vi "HAPS_PhaseGainSweep_Preamp.vi"() -> ()   [LabVIEW 2023, in "HAPS.lvlib"]
uses:
  HAPS.lvlib
  HAPS_SerialPort.ctl
  MCU_Function.ctl
  set_ele.ctl
  HAPS_MCU_ELE_Func.ctl
  R_S/R_S.lvlib
panel:
  out "dup path":path
  out "Phase_step":i32
  out "Gain_step":i32
  out "channel":i32
  out "chain_id":i32
  out "group":i32
  out "array_id":i32
  in  "Gain_Start_Step":i32=16
  in  "Phase Sweep Step":i32=64
  in  "Gain Sweep Step":i32=1
  in  "comn_gain":i32=17
  in  "Init?":bool=TRUE
  in  "File_note":string
  out "Duration(sec)":dbl
  out "In-Phase : Phase(degree)":dbl[](graph)
  out "In-Phase : Gain(dB)":dbl[](graph)
  in  "Phase diff. Criteria":dbl format="%#_13g"
  in  "Tx/Rx":enum16{"Rx", "Tx"}(ring)=enum."Tx"
  in  "array_id (MCU index)":i32
  in  "MCU_UART_addr":refnum<visa-resource-name>="COM8"
  in  "Target(degree)":dbl format="%#_13g"
  in  "SweepPoints":i32=11
  in  "sParameter":i32=21
  in  "Stop_Freq(GHz)":dbl=39.5
  in  "Start_Freq(GHz)":dbl=38.5
  in  "VISA resource name":refnum<visa-resource-name>="TCPIP0::192.168.119.45::inst0::INSTR"
  in  "HAPS_Equipment":enum16{"Keysight", "R&S"}(ring)=enum."R&S"
  # "HAPS_24x24_PhaseGain_Sweep_Preamp_v1.3"
  # "VNA"
  # "DUT"
  # "K:4718\nR:2798"
  # "TCPIP0::192.168.1.31::hislip0::INSTR"
  # "Test Status"
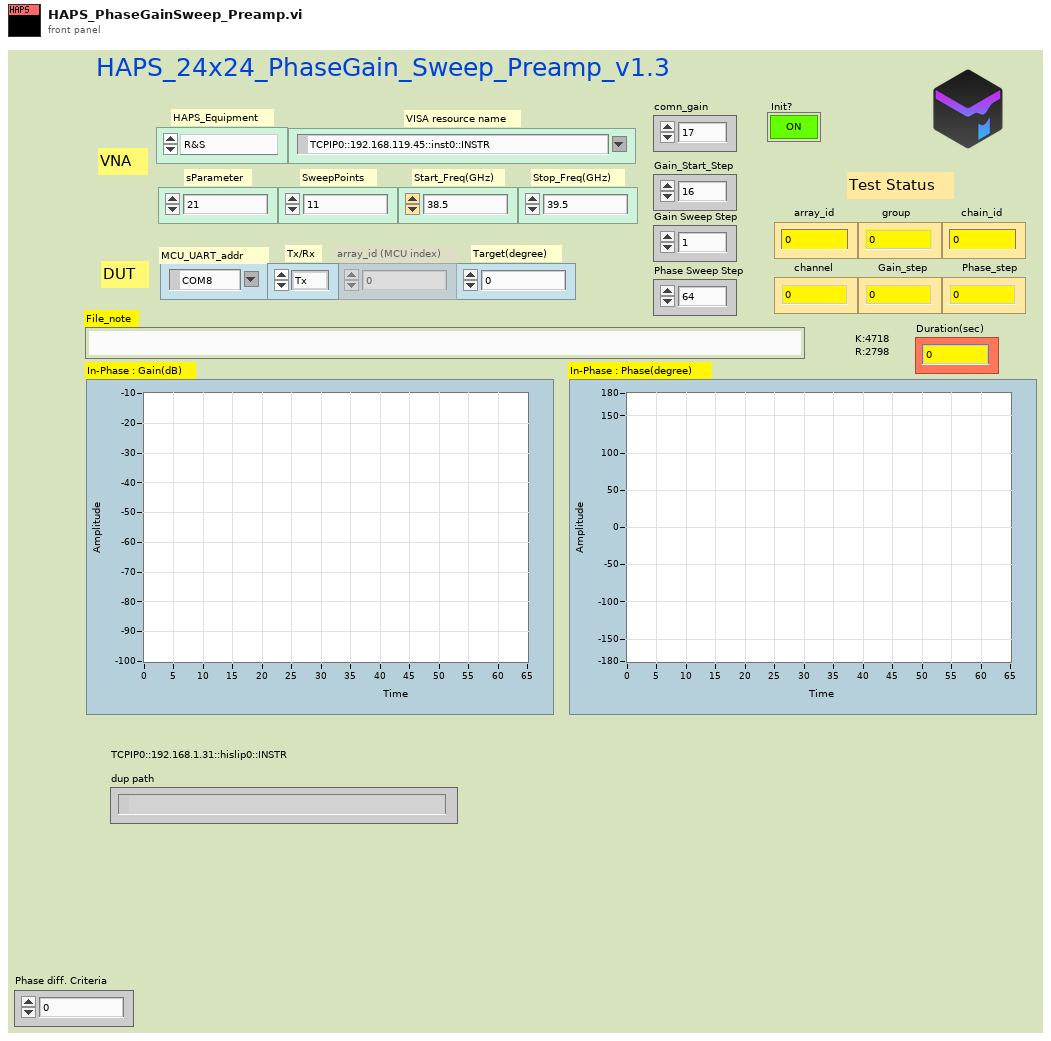
[diagram p1: front panel]
types:
  T1 = typedef "HAPS.lvlib/HAPS_SerialPort.ctl" = enum16{"Init", "Close", "CMD", "Flush"}
  T2 = typedef "HAPS.lvlib/HAPS_MCU_ELE_Func.ctl" = enum16{"array_init", "set_com_gain", "set_ch_gain_phase", "set_pd_range", "get_preamp_temp", "get_bfic_temp", "get_tx_pd", "ch_on", "ch_on_2", "ch_ctrl_all", "array_ctrl_src"}
  T3 = typedef "HAPS.lvlib/MCU_Function.ctl" = cluster{"Tx/Rx":enum16{"Rx", "Tx"}, "Enable?":enum16{"OFF", "On"}, "Source":enum16{"MCU", "ACU"}}
  T4 = typedef "HAPS.lvlib/set_ele.ctl" = cluster{"ch":i32, "chain_id":i32, "group":i32, "array_id":i32, "ele_phase":i32, "ele_gain":i32, "com_gain":i32, "pd_range":i32}
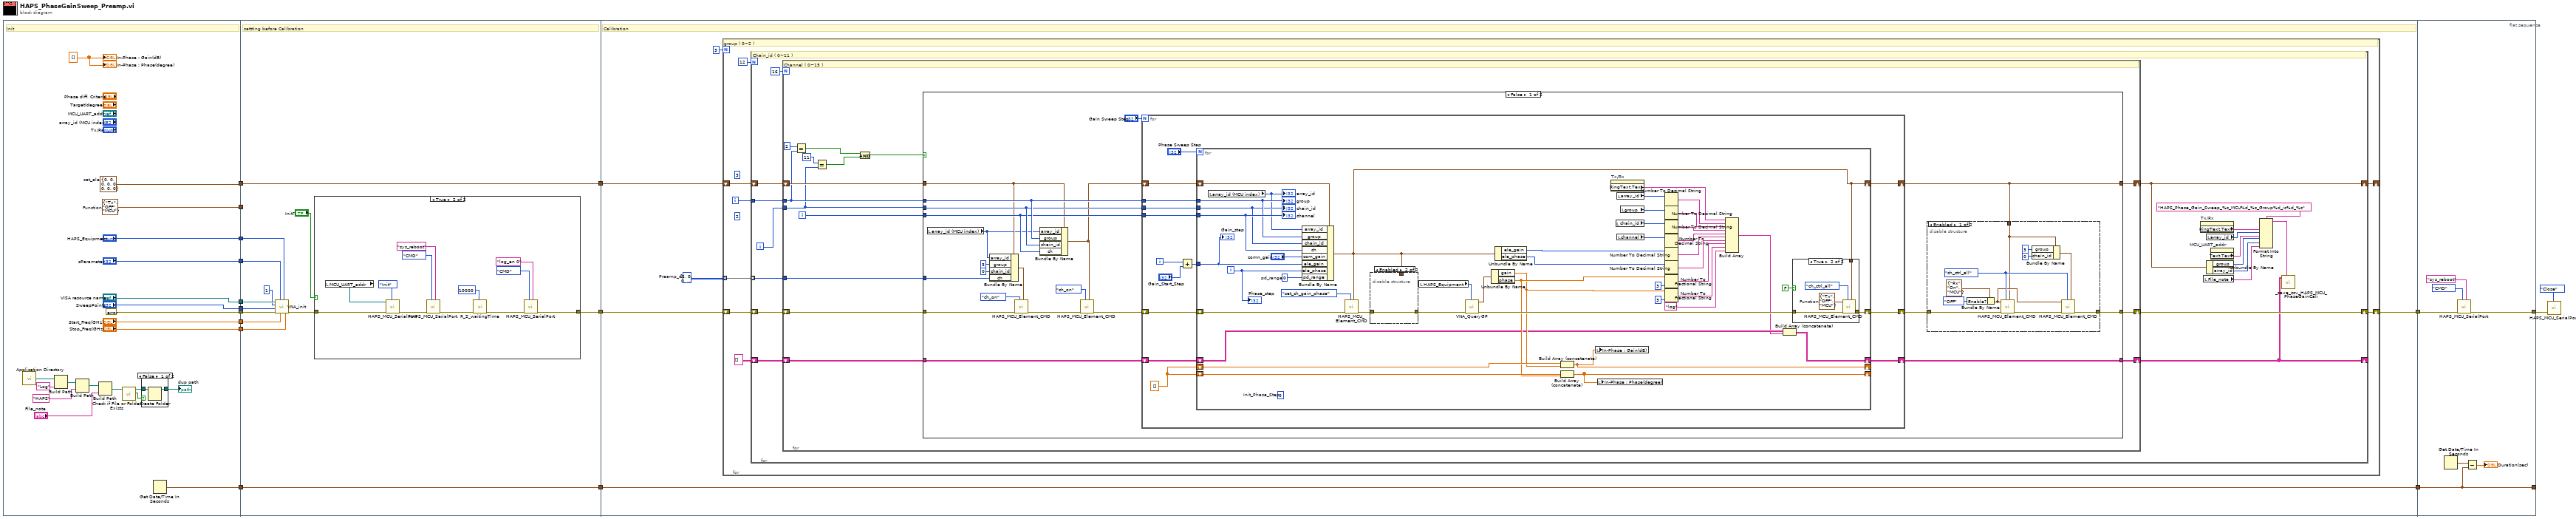
[diagram p0: block diagram]
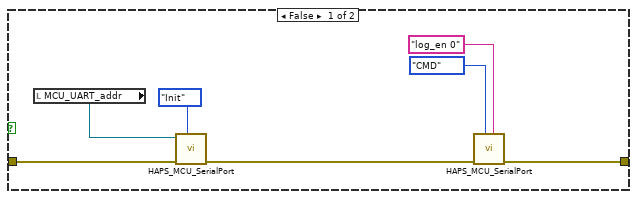
[diagram p3: hidden frame]
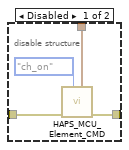
[diagram p4: hidden frame]
diagram:
  n1 = flat-sequence {
    tunnel: [w31] -> w17
    tunnel: [w38] -> w16
    tunnel: [errorcluster {"status"=FALSE, "code"=0, "source"=""} ("error in")] -> w14
    tunnel: ["sParameter"] -> w12
    tunnel: ["VISA resource name"] -> w11
    tunnel: ["Start_Freq(GHz)"] -> w10
    tunnel: ["Stop_Freq(GHz)"] -> w9
    tunnel: ["SweepPoints"] -> w8
    tunnel: ["HAPS_Equipment"] -> w7
    tunnel: [w28] -> w5
    tunnel: w17 -> [w54]
    tunnel: w16 -> [_]
    tunnel: [w54] -> w15
    tunnel: w14 -> [w53]
    tunnel: [w45] -> w13
    tunnel: w12 -> [w52]
    tunnel: w11 -> [w51]
    tunnel: w10 -> [w50]
    tunnel: w9 -> [w49]
    tunnel: w8 -> [w48]
    tunnel: w7 -> [w44]
    tunnel: [w43] -> w6
    tunnel: w5 -> [w43]
    tunnel: w15 -> [w78]
    tunnel: w13 -> [w79]
    tunnel: w6 -> [w76]
    tunnel: [w76] -> w4
    tunnel: [w74] -> w3
    tunnel: [w233] -> _
    tunnel: w4 -> [w233]
    tunnel: w3 -> [w229]
    tunnel: [w228] -> w2
    frame #0 {
      w29 = dbl[] []
      w31 = T4 {"ch"=0, "chain_id"=0, "group"=0, "array_id"=0, "ele_phase"=0, "ele_gain"=0, "com_gain"=0, "pd_range"=0}  # set_ele
      w38 = T3 {"Tx/Rx"=enum."Tx", "Enable?"=enum."OFF", "Source"=enum."MCU"}  # Function
      # "Init"
      n2 = call <vilib>:"Application Directory.vi"() -> ("Application Directory"=w26:path)
      n3 = Build Path(base path=w26, name or relative path="Log") -> (appended path=w27:path)
      n4 = Build Path(base path=w27, name or relative path="HAPS") -> (appended path=w23:path)
      n5 = Build Path(base path=w23, name or relative path="File_note") -> (appended path=w21:path)
      n6 = call <vilib>:"Check if File or Folder Exists.vi"("path"=w21) -> ("file or folder exists?"=w20:bool, "dup path"=w19:path)  [unwired: 8 in, 1 out]
      n7 = case shown="False" w20 {
        tunnel: w19 -> [w40 w41]
        tunnel: [w39 w41] -> w18
        frame False {
          n8 = Create Folder(path (use dialog)=w40) -> (created path=w39:path)  [unwired: 2 in, 2 out]
        }
        frame True {
        }
      }
      "dup path" <- w18
      n9 = Get Date/Time In Seconds() -> (seconds since 1Jan1904=w28:timestamp)
      "In-Phase : Gain(dB)" <- w29
      "In-Phase : Phase(degree)" <- w29
    }
    frame #1 {
      # "settting before Calibration"
      n10 = call "VNA_init.vi"("Stop_Freq(GHz)"=w49, "HAPS_MCU_CMD"=w44, "Start_Freq(GHz)"=w50, "sParameter"=w52, "error in"=w53, "SweepPoints"=w48, "Mark no."=1, "VISA resource name"=w51) -> ("error out"=w46:errorcluster)  [unwired: 3 in]
      n11 = case shown="True" "Init?" {
        tunnel: w46 -> [w58 w71]
        tunnel: [w55 w68] -> w45
        frame False {
          n12 = local read "MCU_UART_addr"() -> (w56:refnum<visa-resource-name>)
          n13 = call "HAPS_MCU_SerialPort.vi"("HAPS_SerialPort_Func"=HAPS_SerialPort."Init", "error in"=w58, "VISA resource name"=w56) -> ("error out"=w59:errorcluster)  [unwired: 6 in, 2 out]
          n14 = call "HAPS_MCU_SerialPort.vi"("Command"="log_en 0", "HAPS_SerialPort_Func"=enum16{"Init", "Close", "CMD"}."CMD" ("HAPS_SerialPort"), "error in"=w59) -> ("error out"=w55:errorcluster)  [unwired: 6 in, 2 out]
        }
        frame True {
          n15 = local read "MCU_UART_addr"() -> (w69:refnum<visa-resource-name>)
          n16 = call "HAPS_MCU_SerialPort.vi"("HAPS_SerialPort_Func"=HAPS_SerialPort."Init", "error in"=w71, "VISA resource name"=w69) -> ("error out"=w65:errorcluster)  [unwired: 6 in, 2 out]
          n17 = call "HAPS_MCU_SerialPort.vi"("Command"="sys_reboot", "HAPS_SerialPort_Func"=enum16{"Init", "Close", "CMD"}."CMD" ("HAPS_SerialPort"), "error in"=w65) -> ("error out"=w64:errorcluster)  [unwired: 6 in, 2 out]
          n18 = call "R_S_waitingTime.vi"("Waiting Time(ms)"=u32 10000, "error in"=w64) -> ("error out"=w63:errorcluster)  [unwired: 9 in]
          n19 = call "HAPS_MCU_SerialPort.vi"("Command"="log_en 0", "HAPS_SerialPort_Func"=enum16{"Init", "Close", "CMD"}."CMD" ("HAPS_SerialPort"), "error in"=w63) -> ("error out"=w68:errorcluster)  [unwired: 6 in, 2 out]
        }
      }
    }
    frame #2 {
      w75 = i32[][] [[2, 0, 0, 8, 8, 10, 11, 9, 9, 1, 1, 3], [3, 1, 1, 9, 9, 11, 13, 15, 15, 7, 7, 5], [5, 7, 7, 15, 15, 13, 14, 14, 6, 6, 4, 12]]  # Preamp_ch
      # "Calibration"
      n20 = for {
        N: 3 -> [_]
        shift-right: [w80] -> _
        shift-left: w78 -> [w85]
        shift-right: [w87] -> w74
        shift-left: w79 -> [w86]
        tunnel: w75 -> [w82] mode=indexing
        i -> [w83]
        (unwired) 2
        (unwired) 3
        # "group ( 0~2 )"
        n21 = for {
          N: 12 -> [_]
          shift-right: [w91] -> w80
          shift-left: w85 -> [w103]
          shift-right: [w88] -> _
          shift-left: string[][] [] -> [w102]
          shift-right: [w99] -> w87
          shift-left: w86 -> [w104]
          tunnel: w83 -> [w101]
          tunnel: w82 -> [w98] mode=indexing
          i -> [w100]
          # "Chain_id ( 0~11 )"
          n22 = for {
            N: 16 -> [_]
            shift-right: [w117] -> w91
            shift-left: w103 -> [w120]
            shift-right: [w115] -> w88
            shift-left: w102 -> [w116]
            shift-right: [w118] -> w99
            shift-left: w104 -> [w119]
            tunnel: w101 -> [w114]
            tunnel: w100 -> [w107]
            tunnel: w98 -> [w106]
            i -> [w108]
            # "Channel ( 0~15 )"
            n23 = Equal?(x=2, y=w114) -> (x = y?=w111:bool)
            n24 = Equal?(x=11, y=w107) -> (x = y?=w110:bool)
            n25 = And(x=w111, y=w110) -> (x .and. y?=w109:bool)
            n26 = case shown="False" w109 {
              tunnel: w120 -> [w129 w226]
              tunnel: w108 -> [w138 _]
              tunnel: w119 -> [w130 w225]
              tunnel: w114 -> [w140 _]
              tunnel: w107 -> [w139 _]
              tunnel: [w134 w225] -> w118
              tunnel: [w133 w226] -> w117
              tunnel: w116 -> [w141 w227]
              tunnel: [w122 w227] -> w115
              tunnel: w106 -> [w124 _]
              frame False {
                n27 = local read "array_id (MCU index)"() -> (w127:i32)
                n28 = Bundle By Name(cluster=w129, "array_id"=w127, "group"=3, "chain_id"=0, "ch"=w124) -> (w128:T4)
                n29 = call "HAPS_MCU_Element_CMD.vi"("set_ele"=w128, "HAPS_MCU_ELE_Func."=HAPS_MCU_ELE_Func."ch_on", "error in"=w130) -> ("error out"=w131:errorcluster)  [unwired: 7 in, 1 out]
                n30 = Bundle By Name(cluster=w129, "array_id"=w127, "group"=w140, "chain_id"=w139, "ch"=w138) -> (w123:T4)
                n31 = call "HAPS_MCU_Element_CMD.vi"("set_ele"=w123, "HAPS_MCU_ELE_Func."=HAPS_MCU_ELE_Func."ch_on", "error in"=w131) -> ("error out"=w136:errorcluster)  [unwired: 7 in, 1 out]
                n32 = for {
                  N: "Gain Sweep Step" -> [_]
                  tunnel: w140 -> [w153]
                  tunnel: w139 -> [w152]
                  tunnel: w138 -> [w151]
                  shift-right: [w149] -> w135
                  shift-left: w136 -> [w150]
                  shift-right: [w148] -> w133
                  shift-left: w123 -> [w147]
                  shift-right: [w146] -> w122
                  shift-left: w141 -> [w154]
                  i -> [w145]
                  w142 = dbl[] []
                  n33 = Add(x=w145, y="Gain_Start_Step") -> (x+y=w144:i32)
                  n34 = for {
                    N: "Phase Sweep Step" -> [_]
                    tunnel: w151 -> [w200]
                    tunnel: w153 -> [w198]
                    tunnel: w152 -> [w197]
                    shift-right: [w178] -> _
                    shift-left: w142 -> [w180]
                    shift-right: [w177] -> _
                    shift-left: w142 -> [w179]
                    shift-right: [w175] -> w149
                    shift-left: w150 -> [w199]
                    shift-right: [w165] -> w148
                    shift-left: w147 -> [w201]
                    shift-right: [w169] -> w146
                    shift-left: w154 -> [w171]
                    tunnel: w144 -> [w157]
                    i -> [w156]
                    w195 = 0  # pd_range
                    (unwired) 0  # Init_Phase_Step
                    n35 = local read "array_id (MCU index)"() -> (w193:i32)
                    "array_id" <- w193
                    n36 = Bundle By Name(cluster=w201, "array_id"=w193, "group"=w198, "chain_id"=w197, "ch"=w200, "com_gain"="comn_gain", "ele_gain"=w157, "ele_phase"=w156, "pd_range"=w195) -> (w165:T4)
                    n37 = call "HAPS_MCU_Element_CMD.vi"("set_ele"=w165, "HAPS_MCU_ELE_Func."=HAPS_MCU_ELE_Func."set_ch_gain_phase", "error in"=w199) -> ("error out"=w167:errorcluster)  [unwired: 7 in, 1 out]
                    n38 = disable-structure shown="Enabled" {
                      disable-tunnel: w167 -> [w205 w206]
                      disable-tunnel: [w204 w206] -> w166
                      disable-tunnel: w165 -> [w202 _]
                      frame Disabled {
                        n39 = call "HAPS_MCU_Element_CMD.vi"("set_ele"=w202, "HAPS_MCU_ELE_Func."=HAPS_MCU_ELE_Func."ch_on", "error in"=w205) -> ("error out"=w204:errorcluster)  [unwired: 7 in, 1 out]
                      }
                      frame Enabled {
                      }
                    }
                    n40 = local read "HAPS_Equipment"() -> (w182:enum16{"Keysight", "R&S"})
                    n41 = call "VNA_QueryGP.vi"("HAPS_Equipment"=w182, "error in"=w166) -> ("error out"=w176:errorcluster, "queryMarker"=w181:cluster{"gain":dbl, "phase":dbl})  [unwired: 8 in]
                    n42 = Unbundle By Name(w181) -> ("gain"=w172:dbl, "phase"=w173:dbl)
                    n43 = Unbundle By Name(w165) -> ("ele_gain"=w158:i32, "ele_phase"=w174:i32)
                    n44 = Build Array (concatenate)(w179, w173) -> (w177:dbl[])
                    n45 = Build Array (concatenate)(w180, w172) -> (w178:dbl[])
                    n46 = local write "In-Phase : Gain(dB)"(w178) -> ()
                    n47 = local write "In-Phase : Phase(degree)"(w177) -> ()
                    n48 = property on="Tx/Rx" class="Enum (strict)"() -> ("RingText.Text"=w159:string)  [unwired: 2 in, 2 out]
                    n49 = local read "chain_id"() -> (w184:i32)
                    n50 = local read "array_id"() -> (w186:i32)
                    n51 = local read "channel"() -> (w183:i32)
                    n52 = local read "group"() -> (w185:i32)
                    n53 = Number To Decimal String(number=w186) -> (decimal integer string=w160:string)  [unwired: 1 in]
                    n54 = Number To Decimal String(number=w185) -> (decimal integer string=w161:string)  [unwired: 1 in]
                    n55 = Number To Decimal String(number=w184) -> (decimal integer string=w162:string)  [unwired: 1 in]
                    n56 = Number To Decimal String(number=w183) -> (decimal integer string=w163:string)  [unwired: 1 in]
                    n57 = Number To Decimal String(number=w158) -> (decimal integer string=w164:string)  [unwired: 1 in]
                    n58 = Number To Decimal String(number=w174) -> (decimal integer string=w187:string)  [unwired: 1 in]
                    n59 = Number To Fractional String(number=w173, precision (6)=i16 3) -> (F-format string=w190:string)  [unwired: 2 in]
                    n60 = Number To Fractional String(number=w172, precision (6)=i16 3) -> (F-format string=w191:string)  [unwired: 2 in]
                    n61 = Build Array(w159, w160, w161, w162, w163, w164, w187, w190, w191, "log") -> (w170:string[])
                    n62 = Build Array (concatenate)(w171, w170) -> (w169:string[][])
                    n63 = case shown="True" FALSE {
                      tunnel: w176 -> [w207 w210]
                      tunnel: [w207 w209] -> w175
                      tunnel: w165 -> [_ w208]
                      frame False {
                      }
                      frame True {
                        w212 = T3 {"Tx/Rx"=enum."Tx", "Enable?"=enum."OFF", "Source"=enum."MCU"}  # Function
                        n64 = call "HAPS_MCU_Element_CMD.vi"("set_ele"=w208, "HAPS_MCU_ELE_Func."=HAPS_MCU_ELE_Func."ch_ctrl_all", "error in"=w210, "Function"=w212) -> ("error out"=w209:errorcluster)  [unwired: 6 in, 1 out]
                      }
                    }
                    "group" <- w198
                    "chain_id" <- w197
                    "channel" <- w200
                    "Gain_step" <- w157
                    "Phase_step" <- w156
                  }
                }
                n65 = disable-structure shown="Enabled" {
                  disable-tunnel: w135 -> [w223 w224]
                  disable-tunnel: [w219 w224] -> w134
                  disable-tunnel: w133 -> [w214 _]
                  frame Enabled {
                    w218 = HAPS_MCU_ELE_Func."ch_ctrl_all" ("HAPS_MCU_ELE_Func.")
                    n66 = Bundle By Name(cluster=T3 {"Tx/Rx"=enum."Rx", "Enable?"=enum."On", "Source"=enum."MCU"} ("Function"), "Enable?"=enum16{"OFF", "On"}."OFF") -> (w217:T3)
                    n67 = call "HAPS_MCU_Element_CMD.vi"("set_ele"=w214, "HAPS_MCU_ELE_Func."=w218, "error in"=w223, "Function"=w217) -> ("error out"=w220:errorcluster)  [unwired: 6 in, 1 out]
                    n68 = Bundle By Name(cluster=w214, "group"=3, "chain_id"=0) -> (w213:T4)
                    n69 = call "HAPS_MCU_Element_CMD.vi"("set_ele"=w213, "HAPS_MCU_ELE_Func."=w218, "error in"=w220, "Function"=w217) -> ("error out"=w219:errorcluster)  [unwired: 6 in, 1 out]
                  }
                  frame Disabled {
                  }
                }
              }
              frame True {
              }
            }
          }
          n70 = property on="Tx/Rx" class="Enum (strict)"() -> ("RingText.Text"=w95:string)  [unwired: 2 in, 2 out]
          n71 = local read "File_note"() -> (w89:string)
          n72 = local read "array_id"() -> (w94:i32)
          n73 = Unbundle By Name(w91) -> ("group"=w93:i32, "array_id"=w90:i32)
          n74 = property on="MCU_UART_addr" class="VISAName"() -> ("Text.Text"=w97:string)  [unwired: 2 in, 2 out]
          n75 = Format Into String(format string="HAPS_Phase_Gain_Sweep_%s_MCU%d_%s_Group%d_ic%d_%s", w95, w94, w97, w93, w90, w89) -> (resulting string=w96:string)  [unwired: 2 in, 1 out]
          n76 = call "_save_csv_HAPS_MCU_PhaseGainCali.vi"("NoteName"=w96, "array in"=w88) -> ()  [unwired: 9 in, 1 out]
        }
      }
    }
    frame #3 {
      n77 = Get Date/Time In Seconds() -> (seconds since 1Jan1904=w234:timestamp)
      n78 = call "HAPS_MCU_SerialPort.vi"("Command"="sys_reboot", "HAPS_SerialPort_Func"=enum16{"Init", "Close", "CMD"}."CMD" ("HAPS_SerialPort"), "error in"=w229) -> ("error out"=w228:errorcluster)  [unwired: 6 in, 2 out]
      n79 = Subtract(x=w234, y=w233) -> (x-y=→"Duration(sec)":dbl)
    }
  }
  n80 = call "HAPS_MCU_SerialPort.vi"("HAPS_SerialPort_Func"=HAPS_SerialPort."Close", "error in"=w2) -> ()  [unwired: 7 in, 3 out]
